vi "Snap from Camera (SubVI).vi"(5 "Colums (Y)":u16, 7 "Rows (X)":u16, 8 "error in (no error)":errorcluster, 9 "Live":bool, 10 "Session In":T1, 11 "Image in":T2) -> (0 "error out":errorcluster, 1 "Image Pixels (U8)":u8[][](array[numeric]), 2 "Session Out":T1, 3 "Image out":T2)   [LabVIEW 2017]
uses:
  <vilib>/vision/Image Controls.llb/IMAQ Image.ctl
  <vilib>/userdefined/High Color/IMAQdx.ctl
  <vilib>/vision/driver/NI_Vision_Acquisition_Software.lvlib
  <vilib>/vision/NI_Vision_Development_Module.lvlib
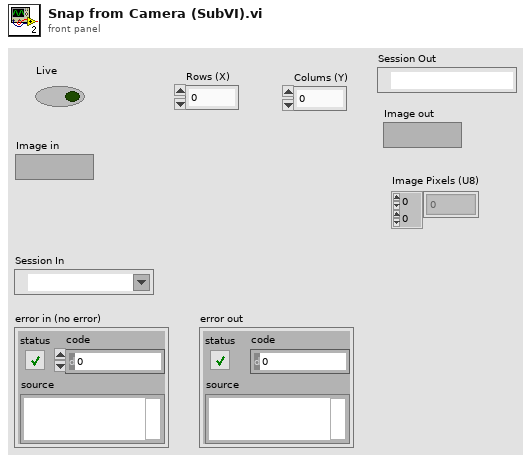
[diagram p1: front panel]
types:
  T1 = typedef "IMAQdx.ctl" = refnum<k21>
  T2 = typedef "IMAQ Image.ctl" = refnum<image>
  T3 = typedef "Image Type" = u32
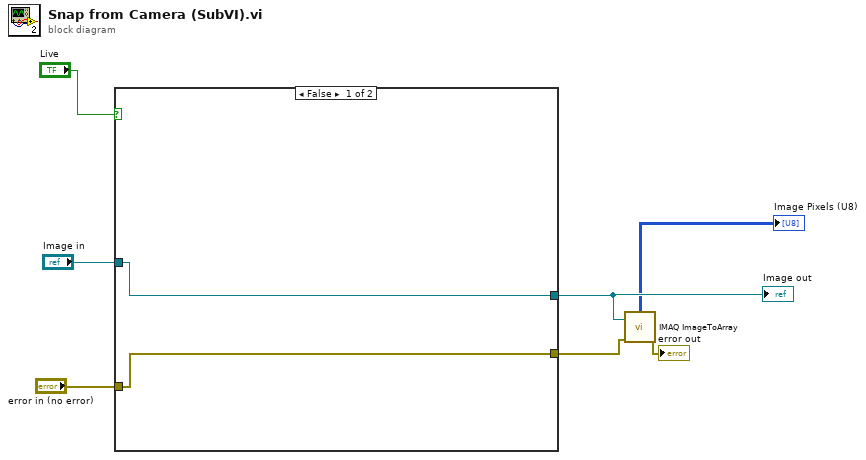
[diagram p0: block diagram]
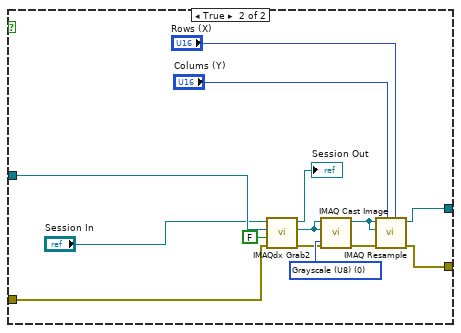
[diagram p2: hidden frame]
diagram:
  n1 = case shown="False" "Live" {
    tunnel: "Image in" -> [w9 w16]
    tunnel: "error in (no error)" -> [w8 w15]
    tunnel: [w8 w10] -> w1
    tunnel: [w9 w11] -> w4
    frame False {
    }
    frame True {
      w19 = T3 0 items=["Grayscale (U8)", "Grayscale (I16)", "Grayscale (SGL)", "Complex (CSG)", "RGB (U32)", "HSL (U32)", "RGB (U64)", "Grayscale (U16)"] ("Image Type")
      n2 = call <vilib>:"IMAQdx Grab2.vi"("error in"=w15, "Wait for Next Buffer? (Yes)"=FALSE, "Image In"=w16, "Session In"="Session In") -> ("error out"=w17:errorcluster, "Image Out"=w18:T2, "Session Out"=→"Session Out":T1)  [unwired: 4 in, 1 out]
      n3 = call "IMAQ Cast Image"("Image Type"=w19, "error in (no error)"=w17, "Image Dst"=w18, "Image Src"=w18) -> ("error out"=w20:errorcluster, "Image Dst Out"=w21:T2)  [unwired: 6 in]
      n4 = call "IMAQ Resample"("X Resolution"="Rows (X)", "Y Resolution"="Colums (Y)", "error in (no error)"=w20, "Image Dst"=w21, "Image Src"=w21) -> ("error out"=w10:errorcluster, "Image Dst Out"=w11:T2)  [unwired: 5 in]
    }
  }
  "Image out" <- w4
  n5 = call "IMAQ ImageToArray"("error in (no error)"=w1, "Image"=w4) -> ("error out"=→"error out":errorcluster, "Image Pixels (U8)"=→"Image Pixels (U8)":u8[][])  [unwired: 2 in, 3 out]
